vi "test_MultipleSessionsReserved_InitializeSession_ReturnsErrorForTooManySessions.vi"(8 "error in":errorcluster) -> (0 "error out":errorcluster, 2 "result":string, 3 "pass":bool)   [LabVIEW 2020, in "MeasurementServerTests.lvlib"]
uses:
  MeasurementServerTests.lvlib
  Helpers/Fake Session Factory/Fake Session Factory.lvclass
  Runtime/MeasurementLink Measurement Server/Helpers/Error Strings Global Internal.vi
  3a947300-8ba6-4980-845e-9b7eeaceb0a3.vi
  Runtime/MeasurementLink Session Management V1/Session Reservation/Initialize and Close Session Behavior.ctl
  Runtime/MeasurementLink Session Management V1/Session Reservation/Session Reservation.lvclass
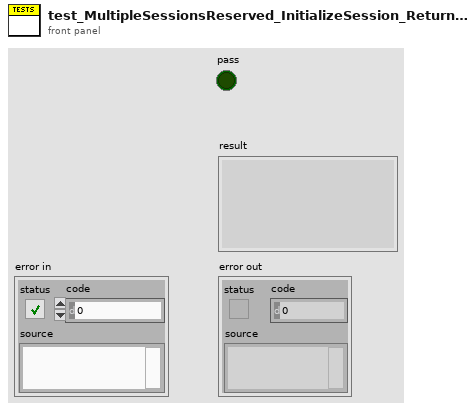
[diagram p1: front panel]
types:
  T1 = typedef "MeasurementLink Session Management V1.lvlib/Session Reservation.lvclass/Initialize and Close Session Behavior.ctl" = enum16{"Auto", "Initialize and Close", "Attach and Detach", "Initialize and Detach", "Attach and Close"}
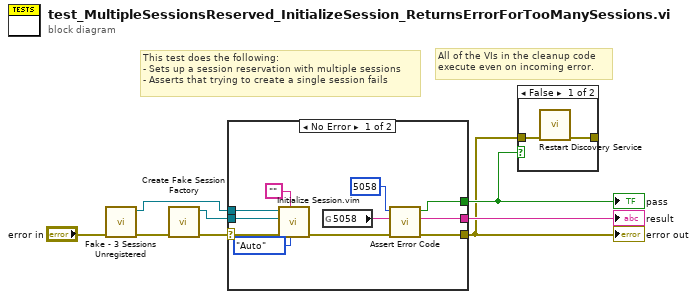
[diagram p0: block diagram]
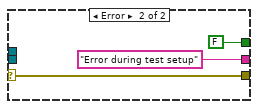
[diagram p2: hidden frame]
diagram:
  # "All of the VIs in the cleanup code\nexecute even on incoming error."
  # "This test does the following:\n- Sets up a session reservation with multiple sessions\n- Asserts that trying to create a single session fails"
  n1 = call "Fake - 3 Sessions Unregistered.vi"("error in"="error in") -> ("error out"=w2:errorcluster, "session reservation out"=w1:refnum<class "Session Reservation.lvclass">)  [unwired: 9 in]
  n2 = call "Create Fake Session Factory.vi"("error in"=w2) -> ("error out"=w5:errorcluster, "fake session factory out"=w4:refnum<class "Fake Session Factory.lvclass">)  [unwired: 9 in]
  n3 = case shown="No Error" w5 {
    selector: w5 -> [w17 w20]
    tunnel: [w11 w20] -> w6
    tunnel: [w15 FALSE] -> w7
    tunnel: [w10 "Error during test setup" ("f")] -> w8
    tunnel: w4 -> [w19 _]
    tunnel: w1 -> [w18 _]
    frame No Error {
      n4 = call "Initialize Session.vim"("initialize and close session behavior"=Initialize_and_Close_Session_Behavior."Auto", "session type"="", "error in"=w17, "session factory"=w19, "session reservation in"=w18) -> ("error out"=w16:errorcluster)  [unwired: 3 in, 3 out]
      n5 = global read "Error Strings Global Internal.vi" "5058"() -> (w12:string)
      n6 = call "Assert Error Code.vi"("error in"=w16, "expected error description"=w12, "expected error code"=5058) -> ("error out"=w11:errorcluster, "details"=w10:string, "error code match?"=w15:bool)  [unwired: 6 in]
    }
    frame Error {
    }
  }
  "error out" <- w6
  "pass" <- w7
  "result" <- w8
  n7 = case shown="False" w7 {
    tunnel: w6 -> [w24 _]
    tunnel: [w23 _] -> _
    frame False {
      n8 = call "Restart Discovery Service.vi"("error in"=w24) -> ("error out"=w23:errorcluster)  [unwired: 10 in]
    }
    frame True {
    }
  }
